vi "SetToneAmplitude.vi"(1 "Selection":u16(ring) items=["Value", "Default", "Minimum", "Maximum"], 2 "Tone Index":u16(ring) items=["Tone 1", "Tone 2", "Tone 3", "Tone 4", "Tone 5", "Tone 6", "Tone 7", "Tone 8", "Tone 9", "Tone 10"], 4 "error in (no error)":errorcluster, 5 "Amplitude[V]":dbl=1.0 format="%#_16g", 6 "ParamWave Name":string, 7 "VISA resource name":refnum<visa-resource-name>) -> (0 "error out":errorcluster, 3 "VISA resource name out":refnum<visa-resource-name>)   [LabVIEW 2020, in "Active Technologies AWG3000.lvlib"]
uses:
  Active Technologies AWG3000.lvlib
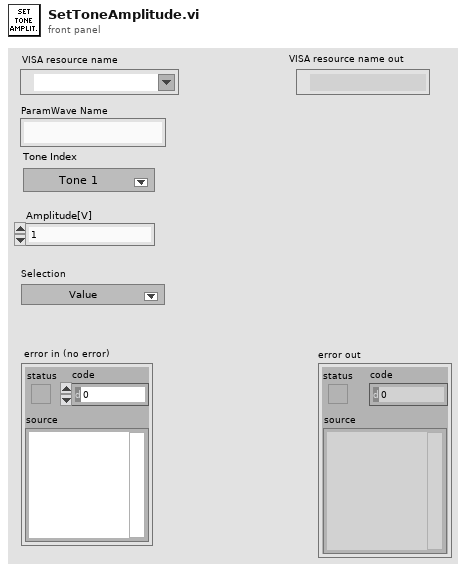
[diagram p1: front panel]
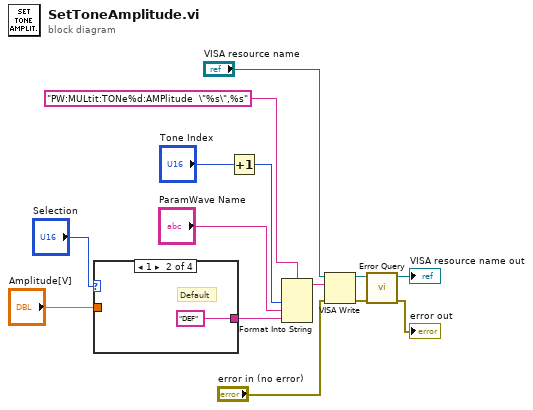
[diagram p0: block diagram]
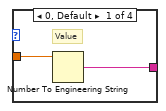
[diagram p2: hidden frame]
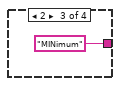
[diagram p3: hidden frame]
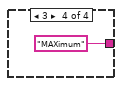
[diagram p4: hidden frame]
diagram:
  n1 = case shown="1" "Selection" {
    tunnel: [w16 "DEF" ("write buffer") "MINimum" ("write buffer") "MAXimum" ("write buffer")] -> w1
    tunnel: "Amplitude[V]" -> [w15 _ _ _]
    frame 0, Default {
      # "Value"
      n2 = Number To Engineering String(4:w15) -> (0:w16:string)  [unwired: 3 in]
    }
    frame 1 {
      # "Default"
    }
    frame 2 {
    }
    frame 3 {
    }
  }
  n3 = Increment(x="Tone Index") -> (x+1=w3:u16)
  n4 = Format Into String(format string="PW:MULtit:TONe%d:AMPlitude  \"%s\",%s" ("write buffer"), w3, "ParamWave Name", w1) -> (resulting string=w6:string)  [unwired: 2 in, 1 out]
  n5 = VISA Write(VISA resource name="VISA resource name", write buffer=w6, error in (no error)="error in (no error)") -> (VISA resource name out=w12:refnum<visa-resource-name>, error out=w11:errorcluster)  [unwired: 1 out]
  n6 = call "Error Query.vi"("error in (no error)"=w11, "VISA resource name"=w12) -> ("error out"=→"error out":errorcluster, "VISA resource name out"=→"VISA resource name out":refnum<visa-resource-name>)  [unwired: 6 in, 2 out]
